vi "Read Skip.vi"(8 "error in (no error)":errorcluster, 11 "StepBase in":refnum<class "Step.lvclass">) -> (0 "error out":errorcluster, 2 "Skip":bool, 3 "StepBase out":refnum<class "Step.lvclass">)   [LabVIEW 2015, in "Step.lvclass"]
uses:
  Step.lvclass
  Step.lvclass/Step.ctl
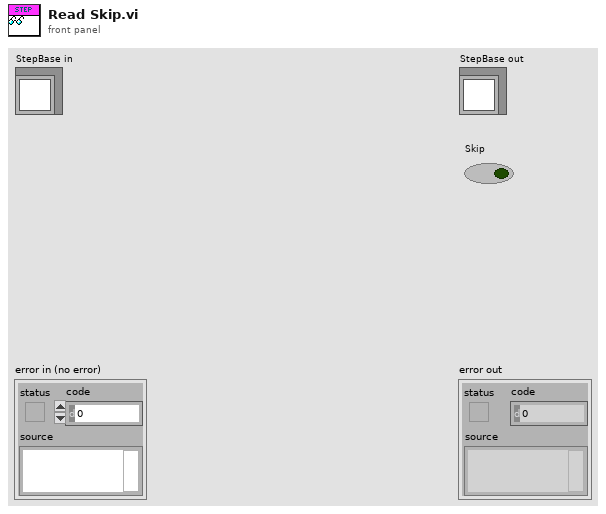
[diagram p1: front panel]
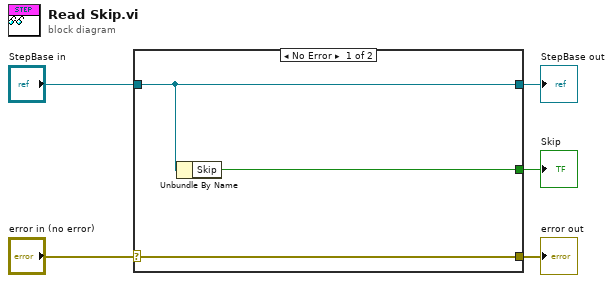
[diagram p0: block diagram]
diagram:
  n1 = case shown="No Error" "error in (no error)" {
    selector: "error in (no error)" -> [w8 w9]
    tunnel: [w8 w9] -> w4
    tunnel: [w7 w10] -> w2
    tunnel: "StepBase in" -> [w7 w10]
    tunnel: [w6 _] -> w1
    frame No Error {
      n2 = Unbundle By Name(w7) -> ("Skip"=w6:bool)
    }
    frame Error {
    }
  }
  "error out" <- w4
  "StepBase out" <- w2
  "Skip" <- w1
